vi "JGP5.vi"() -> ()   [LabVIEW 2019]
doc: "This Vi graphs original values of a 2d array and a squuare root values of the same 2d array\n\nJuan Gamez\nP3600\nCSUSB Physics"
panel:
  out "Data":dbl[][](graph)
  out "Spreadsheet column data":dbl[][](array[numeric])
  out "interval":dbl=1.0
  in  "N intervals":i32=10
  in  "end value":dbl=10.0
  in  "start value":dbl
  # "Juan Gamez\nP3600\nCsusb Physics"
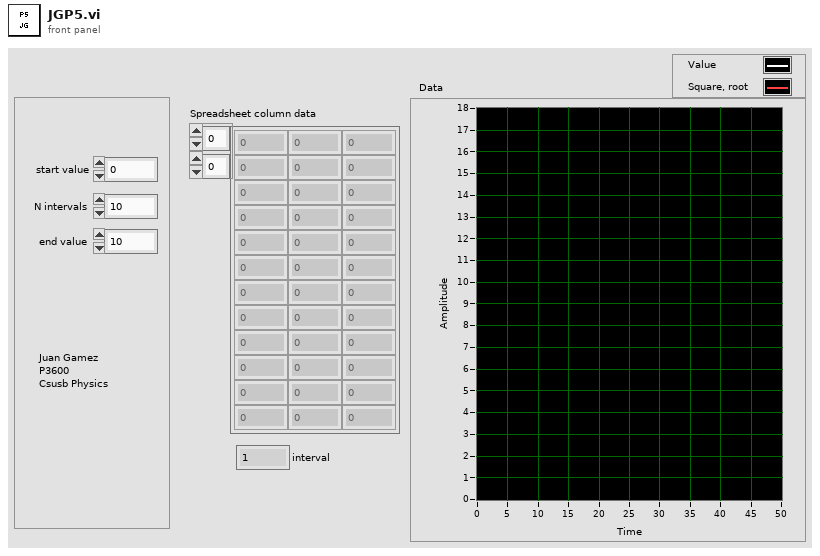
[diagram p1: front panel]
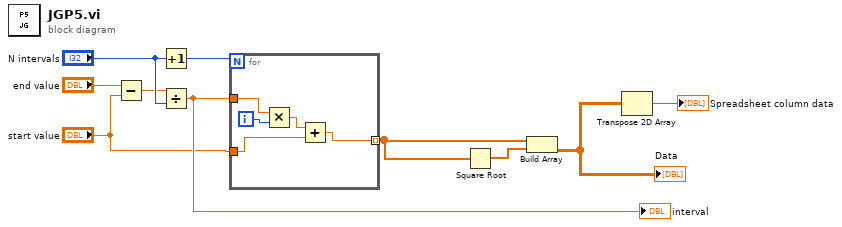
[diagram p0: block diagram]
diagram:
  n1 = Subtract(x="end value", y="start value") -> (x-y=w8:dbl)
  n2 = Increment(x="N intervals") -> (x+1=w7:i32)
  n3 = Divide(x=w8, y="N intervals") -> (x/y=w6:dbl)
  "interval" <- w6
  n4 = for {
    N: w7 -> [_]
    tunnel: w6 -> [w14]
    tunnel: "start value" -> [w12]
    tunnel: [w11] -> w3 mode=indexing
    i -> [w15]
    n5 = Multiply(x=w14, y=w15) -> (x*y=w13:dbl)
    n6 = Add(x=w13, y=w12) -> (x+y=w11:dbl)
  }
  n7 = Square Root(x=w3) -> (sqrt(x)=w4:dbl[])
  n8 = Build Array(w3, w4) -> (w2:dbl[][])
  "Data" <- w2
  n9 = Transpose 2D Array(2D array=w2) -> (transposed array=→"Spreadsheet column data":dbl[][])
